vi "MouseUpCapture.vi"(11 "OrderSelection in":refnum<class "OrderSelection.lvclass">) -> (3 "OrderSelection (dup)":refnum<class "OrderSelection.lvclass">)   [LabVIEW 2020, in "OrderSelection.lvclass"]
uses:
  OrderSelection.lvclass
  <vilib>/Utility/miscctls.llb/LVRectTypeDef.ctl
  OrderSelection.lvclass/OrderSelection.ctl
  <vilib>/Utility/inputDevices.llb/mouseAcquire.vi
  <vilib>/Utility/inputDevices.llb/closeMouse.vi
types:
  T1 = enum32{"Invalid", "Standard", "Closed", "Hidden", "Minimized", "Maximized"}
  T2 = typedef "LVRectTypeDef.ctl" = cluster{"Left":i16, "Top":i16, "Right":i16, "Bottom":i16}
  T3 = typedef "LVAllMonitorsDisplayTypeDef.ctl" = cluster{"Bounds":cluster{"Left":i16, "Top":i16, "Right":i16, "Bottom":i16}, "Depth":i16}[]
  T4 = cluster{"Horizontal":i32, "Vertical":i32, "Scrolling":i32}
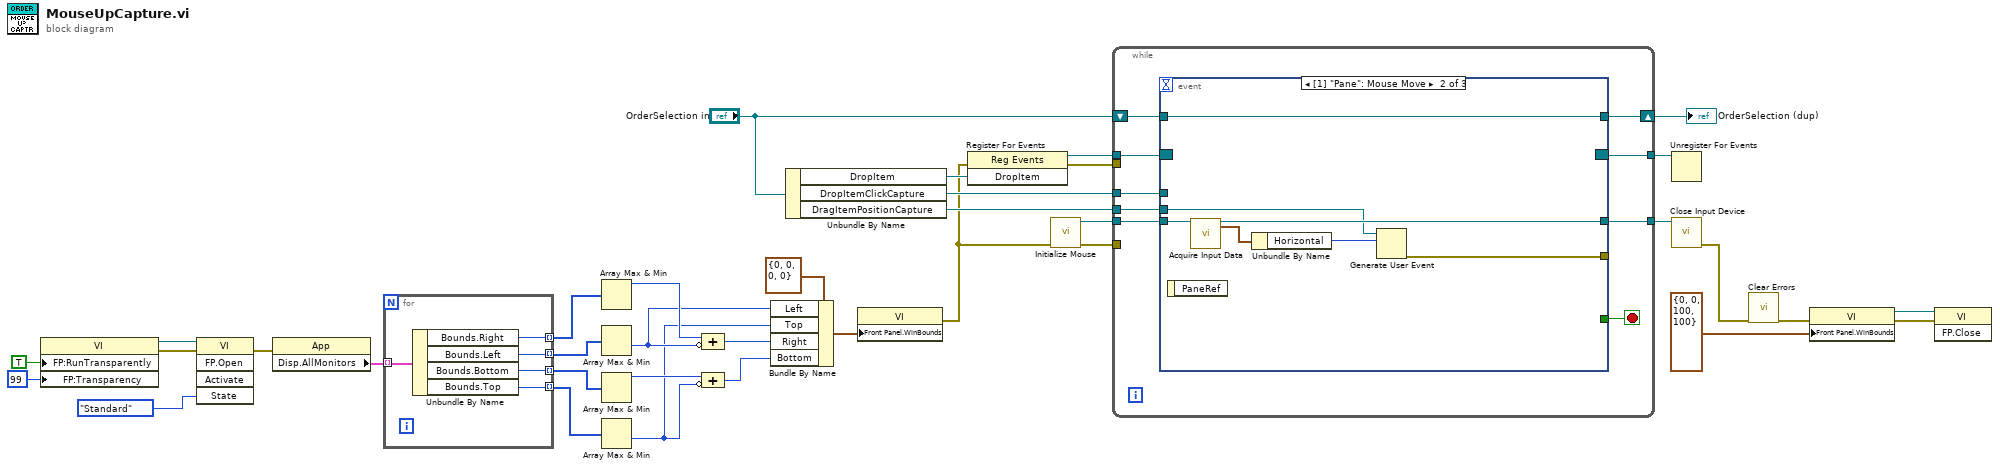
[diagram p0: block diagram]
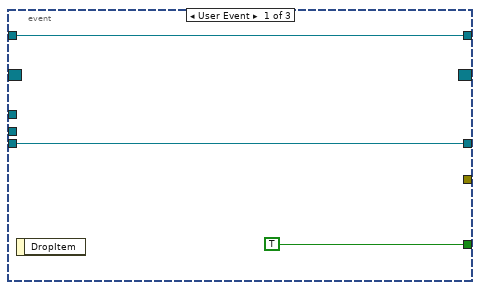
[diagram p2: hidden frame]
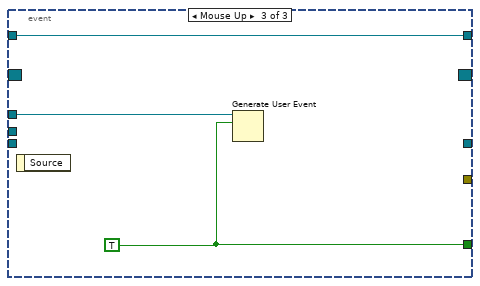
[diagram p3: hidden frame]
diagram:
  n1 = property class="VI"("FP:RunTransparently"=TRUE ("Front Panel Window:Run VI Transparently"), "FP:Transparency"=u8 99 ("Front Panel Window:Transparency")) -> (reference out=w18:refnum<vi>, error out=w17:errorcluster)  [unwired: 2 in]
  n2 = invoke class="VI" method="FP.Open"(reference=w18, error in=w17, "State"=T1."Standard") -> (error out=w15:errorcluster)  [unwired: 2 in, 4 out]
  n3 = property class="App"(error in=w15) -> ("Disp.AllMonitors"=w36:T3)  [unwired: 1 in, 2 out]
  n4 = for {
    tunnel: w36 -> [w41] mode=indexing
    tunnel: [w40] -> w35 mode=indexing
    tunnel: [w39] -> w34 mode=indexing
    tunnel: [w38] -> w33 mode=indexing
    tunnel: [w37] -> w32 mode=indexing
    n5 = Unbundle By Name(w41) -> ("Bounds.Right"=w40:i16, "Bounds.Left"=w39:i16, "Bounds.Bottom"=w38:i16, "Bounds.Top"=w37:i16)
  }
  n6 = Array Max & Min(array=w35) -> (max value=w30:i16)  [unwired: 3 out]
  n7 = Array Max & Min(array=w34) -> (min value=w25:i16)  [unwired: 3 out]
  n8 = Array Max & Min(array=w33) -> (max value=w28:i16)  [unwired: 3 out]
  n9 = Array Max & Min(array=w32) -> (min value=w24:i16)  [unwired: 3 out]
  n10 = Compound Arithmetic op=ADD(w30, invert w25) -> (w29:i16)
  n11 = Compound Arithmetic op=ADD(w28, invert w24) -> (w27:i16)
  n12 = Bundle By Name(cluster=T2 {"Left"=0, "Top"=0, "Right"=0, "Bottom"=0} ("Front Panel Window:Window Bounds"), "Left"=w25, "Top"=w24, "Right"=w29, "Bottom"=w27) -> (w26:T2)
  n13 = Unbundle By Name("OrderSelection in") -> ("DropItem"=w21:refnum<user-event>, "DropItemClickCapture"=w11:refnum<user-event>, "DragItemPositionCapture"=w8:refnum<user-event>)
  n14 = property class="VI"("Front Panel.WinBounds"=w26) -> (error out=w4:errorcluster)  [unwired: 2 in, 1 out]
  n15 = register-events(error in=w4, w21) -> (reference out=w22:refnum<event-registration>, error out=w5:errorcluster)  [unwired: 1 in]
  n16 = call <vilib>:"Initialize Mouse.vi"("error in (no error)"=w4) -> ("error out"=w3:errorcluster, "device ID"=w10:refnum<k1>)  [unwired: 9 in]
  n17 = while {
    tunnel: w22 -> [w49]
    tunnel: w11 -> [w48]
    tunnel: w10 -> [w47]
    tunnel: [w46] -> w9
    tunnel: w8 -> [w45]
    shift-right: [w43] -> w6
    shift-left: "OrderSelection in" -> [w44]
    tunnel: w5 -> [_]
    tunnel: w3 -> [_]
    tunnel: [w42] -> w1
    stop <- w50 stop-if-true
    n18 = event shown="[1] \"Pane\": Mouse Move" {
      selector: w49 -> [_ _ _]
      dyn-events: [_ _ _] -> w42
      timeout: _ -> [_ _ _]
      tunnel: [TRUE _ w63] -> w50
      tunnel: w48 -> [_ _ w62]
      tunnel: w47 -> [w52 w59 _]
      tunnel: [w52 w58 _] -> w46
      tunnel: w45 -> [_ w56 _]
      tunnel: w44 -> [w51 w57 w61]
      tunnel: [w51 w57 w61] -> w43
      tunnel: [_ w54 _] -> _
      event User Event {
        n19 = event-data() -> ()  [unwired: 1 in, 1 out]
      }
      event Mouse Move {
        n20 = event-data() -> ()  [unwired: 1 in, 1 out]
        n21 = call-poly <vilib>:"Acquire Input Data.vi"("device ID"=w59) -> ("device ID"=w58:refnum<k1>, "axis info"=w60:T4)  [unwired: 15 in, 2 out]
        n22 = Unbundle By Name(w60) -> ("Horizontal"=w55:i32)
        n23 = Generate User Event(user event=w56, event data cluster=w55) -> (error out=w54:errorcluster)  [unwired: 2 in, 1 out]
      }
      event Mouse Up {
        w63 = TRUE
        n24 = event-data() -> ()  [unwired: 1 in, 1 out]
        n25 = Generate User Event(user event=w62, event data cluster=w63) -> ()  [unwired: 2 in, 2 out]
      }
    }
  }
  "OrderSelection (dup)" <- w6
  n26 = Unregister For Events(event registration refnum=w1) -> ()  [unwired: 1 in, 1 out]
  n27 = call-poly <vilib>:"Close Input Device.vi"("device ID"=w9) -> ("error out"=w2:errorcluster)  [unwired: 9 in]
  n28 = call <vilib>:"Clear Errors.vi"("error in (no error)"=w2) -> ("error out"=w14:errorcluster)  [unwired: 5 in, 1 out]
  n29 = property class="VI"(error in=w14, "Front Panel.WinBounds"=T2 {"Left"=0, "Top"=0, "Right"=100, "Bottom"=100} ("Front Panel Window:Window Bounds")) -> (reference out=w13:refnum<vi>, error out=w12:errorcluster)  [unwired: 1 in]
  n30 = invoke class="VI" method="FP.Close"(reference=w13, error in=w12) -> ()  [unwired: 1 in, 3 out]
